vi "Get All Processes.vi"(8 "error in (no error)":errorcluster caption="错误输入（无错误）", 11 "ProcessClass 输入":refnum<class "ProcessClass.lvclass"> caption="DNL_LabVIEW Object in") -> (0 "error out":errorcluster caption="错误输出", 2 "Process Names":string[](array[string]), 3 "ProcessClass 输出":refnum<class "ProcessClass.lvclass"> caption="DNL_LabVIEW Object out")   [LabVIEW 2017, in "ProcessClass.lvclass"]
uses:
  ProcessClass.lvclass
  ProcessClass.lvclass/ProcessClass.ctl
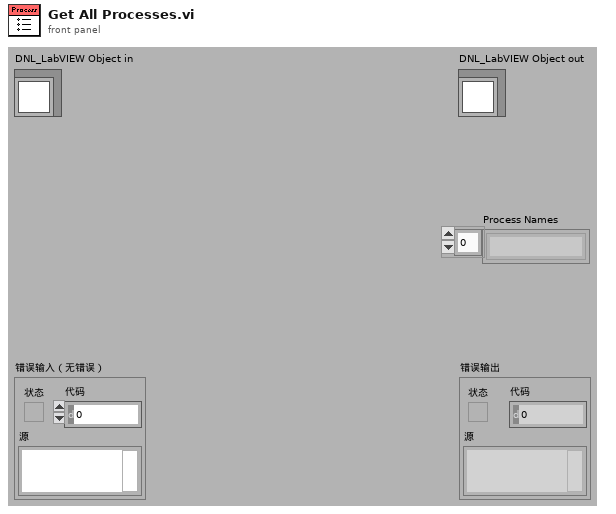
[diagram p1: front panel]
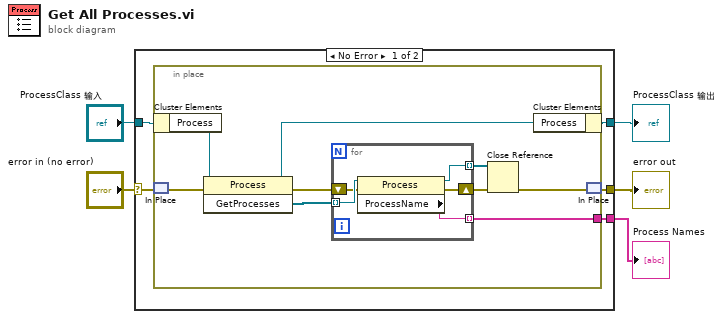
[diagram p0: block diagram]
diagram:
  n1 = case shown="No Error" "error in (no error)" {
    selector: "error in (no error)" -> [w10 w26]
    tunnel: [w9 w26] -> w4
    tunnel: [w7 w25] -> w2
    tunnel: "ProcessClass 输入" -> [w8 w25]
    tunnel: [w6 _] -> w1
    frame No Error {
      n2 = in-place {
        in-place-border: [w14] -> w6
        n3 = in-place-cluster #1(w8) -> ("Process"=w19:refnum<k24>)
        n4 = in-place-match #2(w10) -> (w17:errorcluster)
        n5 = invoke class="Process" method="GetProcesses"(reference=w19, error in=w17) -> (reference out=w18:refnum<k24>, error out=w15:errorcluster, "GetProcesses"=w16:refnum<k24>[])  [unwired: 1 in]
        n6 = for {
          tunnel: w16 -> [w24] mode=indexing
          tunnel: [w23] -> w12 mode=indexing
          tunnel: [w22] -> w14 mode=indexing
          shift-right: [w20] -> w13
          shift-left: w15 -> [w21]
          n7 = property class="Process"(reference=w24, error in=w21) -> (reference out=w23:refnum<k24>, error out=w20:errorcluster, "ProcessName"=w22:string)
        }
        n8 = Close Reference(reference=w12, error in (no error)=w13) -> (error out=w11:errorcluster)
        n9 = in-place-cluster #1("Process"=w18) -> (w7:refnum<class "ProcessClass.lvclass">)
        n10 = in-place-match #2(w11) -> (w9:errorcluster)
      }
    }
    frame Error {
    }
  }
  "error out" <- w4
  "ProcessClass 输出" <- w2
  "Process Names" <- w1
